vi "Time Diff Sub VI.vi"(2 "Start Time (hh:mm:ss)":string, 3 "Start Time Stamp":timestamp, 4 "Current Time (hh:mm:ss)":string, 5 "Current Time Stamp":timestamp) -> (0 "Time Diff (s)":i32, 1 "Time Diff":dbl)   [LabVIEW 2019, in "Mercury iXX.lvlib"]
uses:
  mercury/Mercury iXX.lvlib
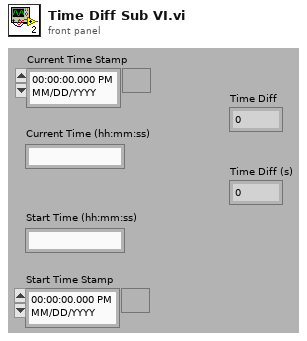
[diagram p1: front panel]
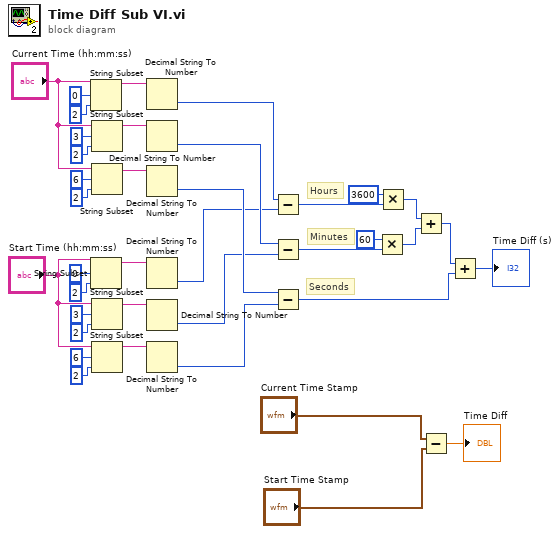
[diagram p0: block diagram]
diagram:
  # "Seconds"
  # "Minutes"
  # "Hours"
  n1 = String Subset(string="Current Time (hh:mm:ss)", offset (0)=0, length (rest)=2 ("length (rest)")) -> (substring=w24:string)
  n2 = String Subset(string="Start Time (hh:mm:ss)", offset (0)=0, length (rest)=2 ("length (rest)")) -> (substring=w21:string)
  n3 = String Subset(string="Current Time (hh:mm:ss)", offset (0)=3, length (rest)=2 ("length (rest)")) -> (substring=w23:string)
  n4 = String Subset(string="Current Time (hh:mm:ss)", offset (0)=6, length (rest)=2 ("length (rest)")) -> (substring=w22:string)
  n5 = String Subset(string="Start Time (hh:mm:ss)", offset (0)=3, length (rest)=2 ("length (rest)")) -> (substring=w20:string)
  n6 = String Subset(string="Start Time (hh:mm:ss)", offset (0)=6, length (rest)=2 ("length (rest)")) -> (substring=w19:string)
  n7 = Decimal String To Number(string=w24) -> (number=w18:i32)  [unwired: 3 out]
  n8 = Decimal String To Number(string=w23) -> (number=w17:i32)  [unwired: 3 out]
  n9 = Decimal String To Number(string=w22) -> (number=w16:i32)  [unwired: 3 out]
  n10 = Decimal String To Number(string=w21) -> (number=w4:i32)  [unwired: 3 out]
  n11 = Decimal String To Number(string=w20) -> (number=w5:i32)  [unwired: 3 out]
  n12 = Decimal String To Number(string=w19) -> (number=w15:i32)  [unwired: 3 out]
  n13 = Subtract(x=w18, y=w4) -> (x-y=w14:i32)
  n14 = Subtract(x=w17, y=w5) -> (x-y=w13:i32)
  n15 = Subtract(x=w16, y=w15) -> (x-y=w7:i32)
  n16 = Multiply(x=60, y=w13) -> (x*y=w10:i32)
  n17 = Multiply(x=3600, y=w14) -> (x*y=w9:i32)
  n18 = Add(x=w9, y=w10) -> (x+y=w8:i32)
  n19 = Subtract(x="Current Time Stamp", y="Start Time Stamp") -> (x-y=→"Time Diff":dbl)
  n20 = Add(x=w8, y=w7) -> (x+y=→"Time Diff (s)":i32)
